vi "setting_height.vi"(9 "Current_height":u32) -> (3 "height_speed":dbl)   [LabVIEW 2015]
panel:
  in  "set_height":u32
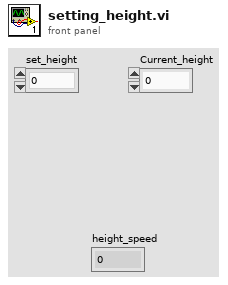
[diagram p1: front panel]
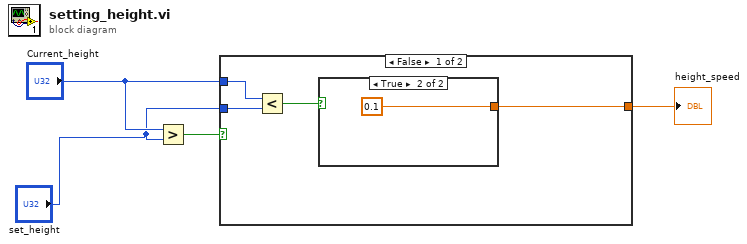
[diagram p0: block diagram]
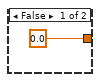
[diagram p2: hidden frame]
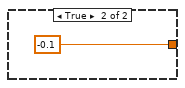
[diagram p3: hidden frame]
diagram:
  n1 = Greater?(x="Current_height", y="set_height") -> (0:w4:bool)
  n2 = case shown="False" w4 {
    tunnel: [w5 -0.1] -> w2
    tunnel: "Current_height" -> [w8 _]
    tunnel: "set_height" -> [w7 _]
    frame False {
      n3 = Less?(x=w8, y=w7) -> (x < y?=w6:bool)
      n4 = case shown="True" w6 {
        tunnel: [sgl 0.0 0.1] -> w5
        frame False {
        }
        frame True {
        }
      }
    }
    frame True {
    }
  }
  "height_speed" <- w2
